vi "Линейка (SubVI).vi"(0 "Mouse ID in":refnum<k1>, 2 "VI reference":refnum<vi>, 5 "error in (no error)":errorcluster) -> (14 "Mouse ID out":refnum<k1>, 16 "Slide Horizontal":u8, 17 "Slide Vertical":u8, 19 "error out":errorcluster)   [LabVIEW 2015]
doc: "Линейка - отрисовывание текущего положения курсора \n в системе координат мишеней"
uses:
  <vilib>/Utility/inputDevices.llb/mouseAcquire.vi
panel:
  out "Mouse on Pane pos Vertical":u32
  out "Mouse on Pane pos Horizontal":u32
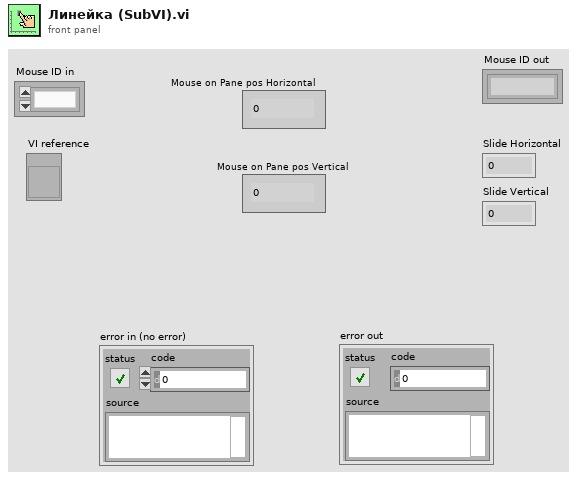
[diagram p1: front panel]
types:
  T1 = typedef "LVRectTypeDef.ctl" = cluster{"Left":i16, "Top":i16, "Right":i16, "Bottom":i16}
  T2 = cluster{"Horizontal":i32, "Vertical":i32, "Scrolling":i32}
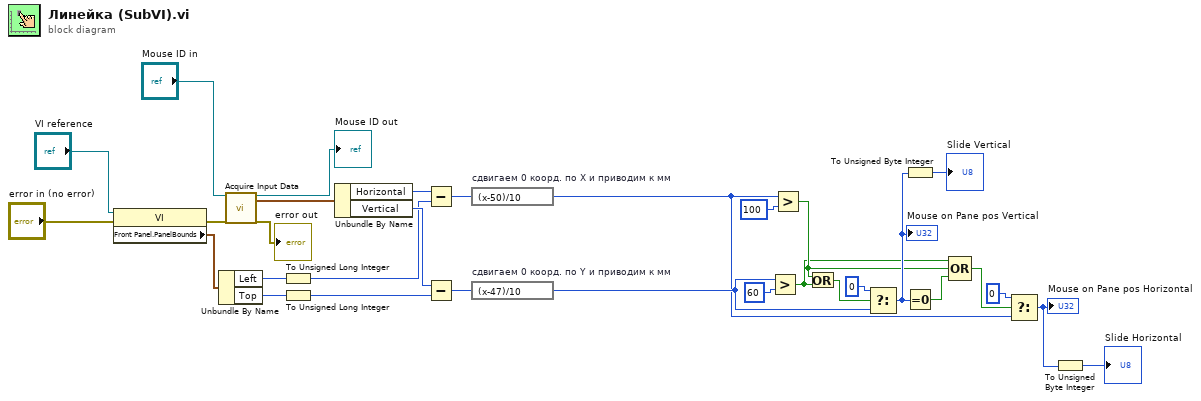
[diagram p0: block diagram]
diagram:
  n1 = property class="VI"(reference="VI reference", error in="error in (no error)") -> (error out=w31:errorcluster, "Front Panel.PanelBounds"=w7:T1)  [unwired: 1 out]
  n2 = Unbundle By Name(w7) -> ("Left"=w8:i16, "Top"=w9:i16)
  n3 = call-poly <vilib>:"Acquire Input Data.vi"("device ID"="Mouse ID in", "error in (no error)"=w31) -> ("device ID"=→"Mouse ID out":refnum<k1>, "axis info"=w5:T2, "error out"=→"error out":errorcluster)  [unwired: 1 in, 14 out]
  n4 = To Unsigned Long Integer(number=w8) -> (unsigned 32bit integer=w11:u32)
  n5 = To Unsigned Long Integer(number=w9) -> (unsigned 32bit integer=w13:u32)
  n6 = Unbundle By Name(w5) -> ("Horizontal"=w12:i32, "Vertical"=w14:i32)
  n7 = Subtract(x=w12, y=w11) -> (x-y=w15:u32)
  n8 = Subtract(x=w14, y=w13) -> (x-y=w16:u32)
  n9 = expression code="(x-50)/10" "сдвигаем 0 коорд. по X и приводим к мм"(w15) -> (w21:u32)
  n10 = expression code="(x-47)/10" "сдвигаем 0 коорд. по Y и приводим к мм"(w16) -> (w22:u32)
  n11 = Greater?(x=w22, y=u32 60) -> (0:w24:bool)
  n12 = Greater?(x=w21, y=u32 100) -> (0:w25:bool)
  n13 = Or(x=w25, y=w24) -> (x .or. y?=w23:bool)
  n14 = Select(t=0, s=w23, f=w22) -> (s? t:f=w28:u32)
  "Mouse on Pane pos Vertical" <- w28
  n15 = To Unsigned Byte Integer(number=w28) -> (unsigned 8bit integer=→"Slide Vertical":u8)
  n16 = Equal To 0?(x=w28) -> (x = 0?=w26:bool)
  n17 = Compound Arithmetic op=OR(w24, w25, w26) -> (w27:bool)
  n18 = Select(t=0, s=w27, f=w21) -> (s? t:f=w29:u32)
  "Mouse on Pane pos Horizontal" <- w29
  n19 = To Unsigned Byte Integer(number=w29) -> (unsigned 8bit integer=→"Slide Horizontal":u8)
